vi "setSlitWidth.vi"(8 "error in (no error)":errorcluster, 10 "position":T1, 11 "MonoCommunicator in":refnum<class "MonoCommunicator.lvclass">) -> (0 "error out":errorcluster, 3 "MonoCommunicator out":refnum<class "MonoCommunicator.lvclass">)   [LabVIEW 2016, in "MonoCommunicator.lvclass"]
uses:
  MonoCommunicator.lvclass
  Typedefs/slit.ctl
  Typedefs/SlitType.ctl
  Typedefs/slitWidth.ctl
  MonoCommunicator.lvclass/MonoCommunicator.ctl
  MonoPubSubData/MonoPubSubData.lvclass/MonoPubSubData.ctl
  MonoPubSubData/MonoPubSubData.lvclass
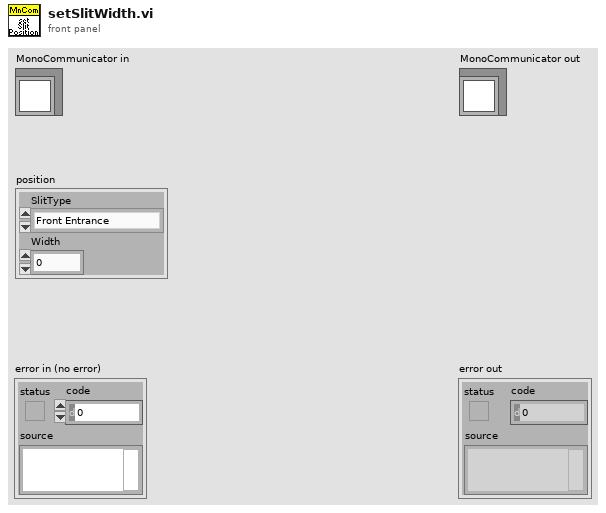
[diagram p1: front panel]
types:
  T1 = typedef "slit.ctl" = cluster{"SlitType":T2, "Width":T3}
  T2 = typedef "SlitType.ctl" = enum16{"Front Entrance", "Side Entrance", "Front Exit", "Side Exit", "First Intermediate", "Second Intermediate"}
  T3 = typedef "slitWidth.ctl" = dbl
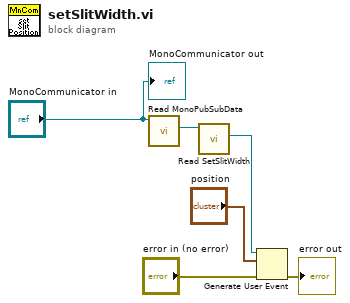
[diagram p0: block diagram]
diagram:
  n1 = call "Read MonoPubSubData.vi"("MonoCommunicator in"="MonoCommunicator in") -> ("MonoPubSubData.lvclass"=w5:refnum<class "MonoPubSubData.lvclass">)  [unwired: 8 in, 2 out]
  n2 = call "Read SetSlitWidth.vi"("MonoPubSubData in"=w5) -> ("SetSlitPosition"=w3:refnum<user-event>)  [unwired: 8 in, 2 out]
  n3 = Generate User Event(user event=w3, event data cluster="position", error in="error in (no error)") -> (error out=→"error out":errorcluster)  [unwired: 1 in, 1 out]
  "MonoCommunicator out" <- "MonoCommunicator in"
